vi "Y5140_SetVolt.vi"(8 "error in (no error)":errorcluster caption="错误输入（无错误）", 11 "MyIndex":u8) -> (0 "error out":errorcluster caption="错误输出", 1 "T/F":bool, 2 "Value":sgl)   [LabVIEW 2015]
uses:
  <vilib>/Instr/_visa.llb/VISA Configure Serial Port (Instr).vi
panel:
  out "VISA":refnum<visa-resource-name> caption="VISA资源名称输出"
  out "Rx":string
  in  "设置电压值(V)":dbl=1.0
  out "Tx":string
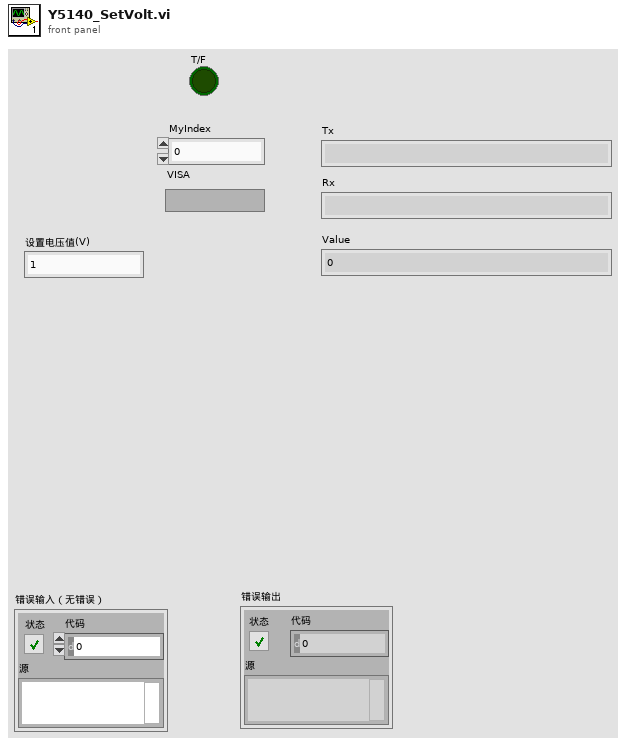
[diagram p1: front panel]
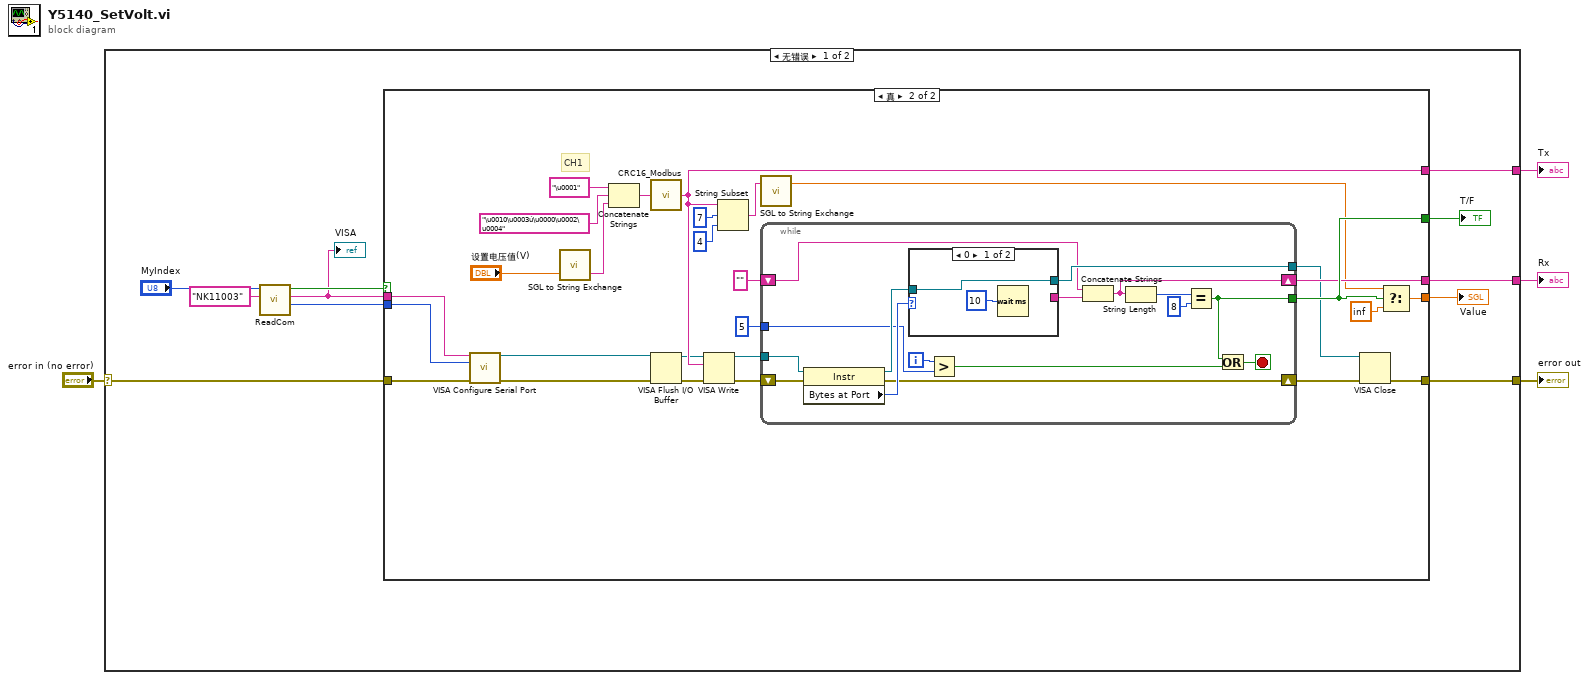
[diagram p0: block diagram]
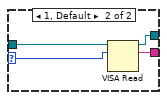
[diagram p3: hidden frame]
diagram:
  n1 = case shown="无错误" "error in (no error)" {
    selector: "error in (no error)" -> [w13 w67]
    tunnel: [w12 w67] -> w3
    tunnel: [w11 _] -> w2
    tunnel: [w10 _] -> w1
    frame No Error {
      n2 = call "ReadCom.vi"("仪器名称"="NK11003", "MyIndex"="MyIndex") -> ("Baudrate"=w5:i32, "COM"=w6:string, "OK?"=w7:bool)  [unwired: 7 in]
      "VISA" <- w6
      n3 = case shown="真" w7 {
        tunnel: [_ w44] -> w15
        tunnel: [_ w43] -> w14
        tunnel: w13 -> [w16 w42]
        tunnel: [w16 w18] -> w12
        tunnel: [_ w40] -> w11
        tunnel: [_ w38] -> w10
        tunnel: w6 -> [_ w21]
        tunnel: w5 -> [_ w20]
        frame False {
        }
        frame True {
          # "CH1"
          n4 = call-poly "VISA Configure Serial Port"("VISA resource name"=w21, "baud rate (9600)"=w20, "error in (no error)"=w42) -> ("VISA resource name out"=w19:refnum<visa-resource-name>, "error out"=w22:errorcluster)  [unwired: 11 in]
          n5 = call "SGL to String Exchange.vi"("SGL In"="设置电压值(V)") -> ("4字节字符串"=w23:string)  [unwired: 1 in, 1 out]
          n6 = Concatenate Strings("\u0001", "\u0010\u0003ú\u0000\u0002\u0004", w23) -> (w24:string)
          n7 = call "CRC16_Modbus.vi"("需要校验的数据"=w24) -> ("String+CRC16"=w40:string)
          n8 = VISA Flush I/O Buffer(VISA resource name=w19, error in (no error)=w22) -> (VISA resource name out=w36:refnum<visa-resource-name>, error out=w35:errorcluster)  [unwired: 1 in]
          n9 = VISA Write(VISA resource name=w36, write buffer=w40, error in (no error)=w35) -> (VISA resource name out=w34:refnum<visa-resource-name>, error out=w33:errorcluster)  [unwired: 1 out]
          n10 = String Subset(string=w40, offset (0)=7 ("偏移量(0)"), length (rest)=4 ("长度（剩余）")) -> (substring=w28:string)
          n11 = call "SGL to String Exchange.vi"("4字节字符串"=w28) -> ("IEE754Floatout"=w27:sgl)  [unwired: 1 in, 1 out]
          n12 = while {
            tunnel: w34 -> [w60]
            tunnel: [w57] -> w17
            shift-right: [w49] -> w38
            shift-left: "" -> [w55]
            tunnel: 5 ("y") -> [w53]
            tunnel: [w45] -> w44
            shift-right: [w51] -> w41
            shift-left: w33 -> [w52]
            i -> [w54]
            stop <- w46 stop-if-true
            n13 = property class="Instr"(reference=w60, error in=w52) -> (reference out=w58:refnum<visa-resource-name>, error out=w51:errorcluster, "Bytes at Port"=w59:u32)
            n14 = case shown="0" w59 {
              selector: w59 -> [_ w65]
              tunnel: w58 -> [w62 w66]
              tunnel: [w62 w64] -> w57
              tunnel: [_ w63] -> w56
              frame 0 {
                n15 = Wait (ms)(milliseconds to wait=u32 10 ("等待时间（毫秒）")) -> ()  [unwired: 1 out]
              }
              frame 1, Default {
                n16 = VISA Read(VISA resource name=w66, byte count=w65) -> (VISA resource name out=w64:refnum<visa-resource-name>, read buffer=w63:string)  [unwired: 1 in, 2 out]
              }
            }
            n17 = Greater?(x=w54, y=w53) -> (0:w50:bool)
            n18 = Concatenate Strings(w55, w56) -> (w49:string)
            n19 = String Length(string=w49) -> (length=w48:i32)
            n20 = Equal?(x=w48, y=8) -> (x = y?=w45:bool)
            n21 = Or(x=w45, y=w50) -> (x .or. y?=w46:bool)
          }
          n22 = VISA Close(VISA resource name=w17, error in (no error)=w41) -> (error out=w18:errorcluster)
          n23 = Select(t=w27, s=w44, f=sgl inf) -> (s? t:f=w43:sgl)
        }
      }
      "T/F" <- w15
      "Value" <- w14
    }
    frame Error {
    }
  }
  "error out" <- w3
  "Tx" <- w2
  "Rx" <- w1
